vi "Display Load Menu Add.vi"(5 "Save":bool=TRUE, 7 "Code Chunk":string, 8 "error in":errorcluster, 9 "Display Name":string, 10 "Node In":string, 11 "VISA resource name":refnum<visa-resource-name>) -> (0 "error out":errorcluster, 2 "Node Out":string, 3 "VISA resource name out":refnum<visa-resource-name>, 4 "Command String":string)   [LabVIEW 2018, in "Keithley 2600 Series.lvlib"]
doc: "This VI will add an entry to the \"USER TESTS\" submenu of the \"LOAD TEST\" menu. Use this VI to make loaded scripts accessible from the front panel.\n\n<b>Functions and Attributes Used</b>\ndisplay.loadmenu.add()"
uses:
  Keithley 2600 Series.lvlib
  Private/GlobalVariables.vi
panel:
  # "(c) 2008 Keithley Instruments, Inc.  ALL RIGHTS RESERVED."
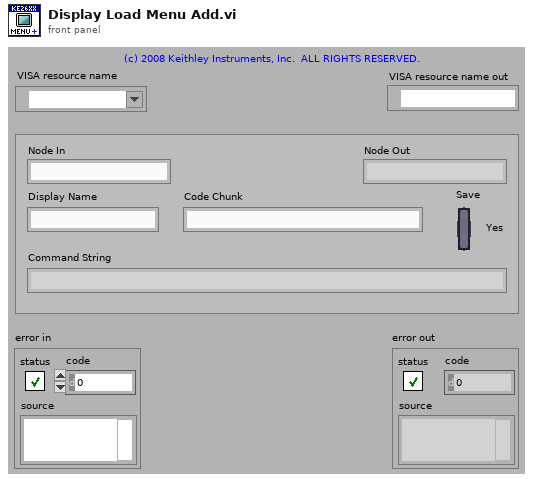
[diagram p1: front panel]
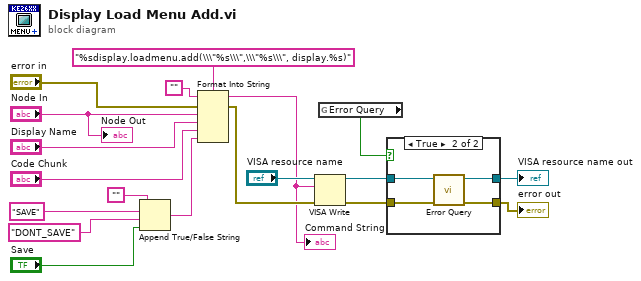
[diagram p0: block diagram]
diagram:
  n1 = Append True/False String(1:"Save", 2:"DONT_SAVE" ("false string"), 3:"SAVE" ("true string"), 4:"") -> (0:w13:string)
  n2 = Format Into String(format string="%sdisplay.loadmenu.add(\\\"%s\\\",\\\"%s\\\", display.%s)", initial string="", error in="error in", "Node In", "Display Name", "Code Chunk", w13) -> (resulting string=w1:string, error out=w8:errorcluster)
  "Command String" <- w1
  n3 = VISA Write(VISA resource name="VISA resource name", write buffer=w1, error in (no error)=w8) -> (VISA resource name out=w5:refnum<visa-resource-name>, error out=w4:errorcluster)  [unwired: 1 out]
  n4 = global read "GlobalVariables.vi" "Error Query"() -> (w6:bool)
  n5 = case shown="True" w6 {
    tunnel: w5 -> [w21 w25]
    tunnel: w4 -> [w20 w24]
    tunnel: [w21 w23] -> w2
    tunnel: [w20 w22] -> w3
    frame False {
    }
    frame True {
      n6 = call "Error Query.vi"("error in (no error)"=w24, "VISA resource name"=w25) -> ("error out"=w22:errorcluster, "VISA resource name out"=w23:refnum<visa-resource-name>)  [unwired: 8 out]
    }
  }
  "VISA resource name out" <- w2
  "error out" <- w3
  "Node Out" <- "Node In"
